vi "AlliGator Simulate Average Lifetime of Linear Combination.vi"(6 "seed":i32=-1, 8 "Error In":errorcluster, 10 "Phasor Parameters":T2, 11 "Simulation Parameters":T1) -> (0 "Error Out":errorcluster, 1 "Average Lifetimes SDV (AlliGator)":dbl[](array[numeric]), 2 "Average Lifetimes (AlliGator)":dbl[](array[numeric]), 3 "Average Lifetimes (Pure Poisson)":dbl[](array[numeric]), 4 "Message":string)   [LabVIEW 2021, in "AlliGator Shot Noise Influence on Average Lifetime.lvlib"]
doc: "Performs the simulations used in the Shot Noise Influence on Average Lifetime tool."
uses:
  AlliGator Shot Noise Influence on Average Lifetime.lvlib
  AlliGator Phasor Simulation Parameters.ctl
  AlliGator Statistics Simulation Parameters.ctl
  Histograms/Linear Histogram Options.ctl
  Histograms/Histogram Bin Option.ctl
  Histograms/Histogram Bin Position.ctl
  Phasor/Phasor Standard Deviation Options.ctl
  31c4b014-1b65-420e-a38b-b52167726bae.vi
  68577856-4cee-4ba6-b73b-a44c9001cbe5.vi
  bd7c4987-2098-4f57-a2c0-f8c7a02182c5.vi
  465ebc7b-c58a-47d8-872f-cf9e5fe3166b.vi
  bd7c4987-2098-4f57-a2c0-f8c7a02182c5.vi/e021cd17-e000-4244-b7f4-ec50548bdfcb.vi
  bd7c4987-2098-4f57-a2c0-f8c7a02182c5.vi/b1828c6e-eb0a-43e9-a724-8b596c52e435.vi
  bd7c4987-2098-4f57-a2c0-f8c7a02182c5.vi/7a6138ed-c001-4311-b538-9ba42ae7c7b1.vi
  bd7c4987-2098-4f57-a2c0-f8c7a02182c5.vi/52c6b4fa-501b-4af0-803b-8bab516ca5d3.vi
  bd7c4987-2098-4f57-a2c0-f8c7a02182c5.vi/d7237e10-35ab-4bcb-a0c6-4883c3f4c990.vi
  bd7c4987-2098-4f57-a2c0-f8c7a02182c5.vi/5fb5dd96-3b97-4592-ba56-58181c8e7105.vi
  bd7c4987-2098-4f57-a2c0-f8c7a02182c5.vi/8e13a849-a393-4484-9968-4af7b25c38d7.vi
  AlliGator Abort.vi
  <userlib>/_OpenG.lib/array/array.llb/Filter 1D Array__ogtk.vi
  <userlib>/_OpenG.lib/array/array.llb/Filter 1D Array (DBL)__ogtk.vi
  <userlib>/_OpenG.lib/array/array.llb/Delete Elements from Array__ogtk.vi
  <userlib>/_OpenG.lib/array/array.llb/Delete Elements from 1D Array (DBL)__ogtk.vi
  <vilib>/Utility/error.llb/Error Cluster From Error Code.vi
  Phasor/Phasor.lvlib
  Histograms/Histogram Window.lvlib
  Math/Math.lvlib
  GUI/GUI.lvlib
  AlliGator Globals, Variables & Constants.lvlib
  Time/Time.lvlib
  Variant/Variant.lvlib
  Utilities/Utilities.lvlib
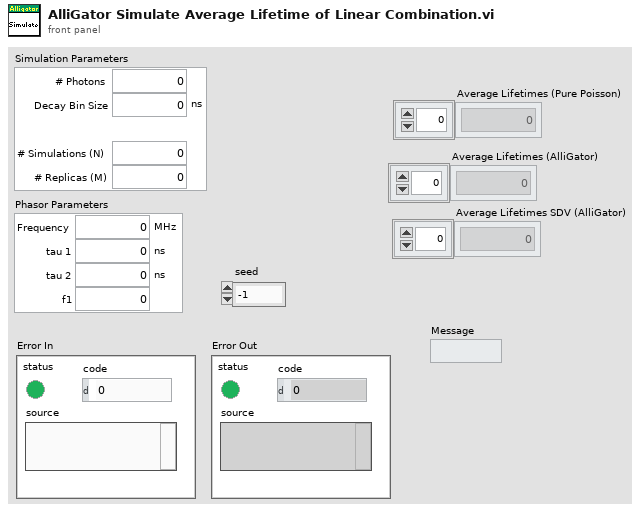
[diagram p1: front panel]
types:
  T1 = typedef "AlliGator Shot Noise Influence on Average Lifetime.lvlib/AlliGator Statistics Simulation Parameters.ctl" = cluster{"# Photons":i32, "# Replicas (M)":i32, "# Simulations (N)":i32, "Decay Bin Size":dbl[unit]}
  T2 = typedef "AlliGator Shot Noise Influence on Average Lifetime.lvlib/AlliGator Phasor Simulation Parameters.ctl" = cluster{"tau 1":dbl[unit], "tau 2":dbl[unit], "f1":dbl, "Frequency":dbl[unit]}
  T3 = typedef "Phasor.lvlib/Phasor Standard Deviation Options.ctl" = cluster{"Compute Estimated SDV":bool, "# Replicas":u32, "Use Estimated Average Phasor":bool}
  T4 = typedef "Histogram Window.lvlib/Linear Histogram Options.ctl" = cluster{"Bin Size":dbl, "Bin Number":i32, "Bin Option":T5, "Min Value":dbl, "Max Value":dbl, "Filter NaN & Infinite Values":bool, "Frequency Plot":bool, "Align Bins":bool, "Bin Location":T6, "Project Outside Values":bool, "Max Histogram Size":i32}
  T5 = typedef "Histogram Window.lvlib/Histogram Bin Option.ctl" = enum32{"Bin Number", "Bin Size"}
  T6 = typedef "Histogram Window.lvlib/Histogram Bin Position.ctl" = enum16{"Left", "Center", "Right"}
  T7 = typedef "Phasor.lvlib/Phasor (g, s).ctl" = cluster{"g":dbl, "s":dbl}
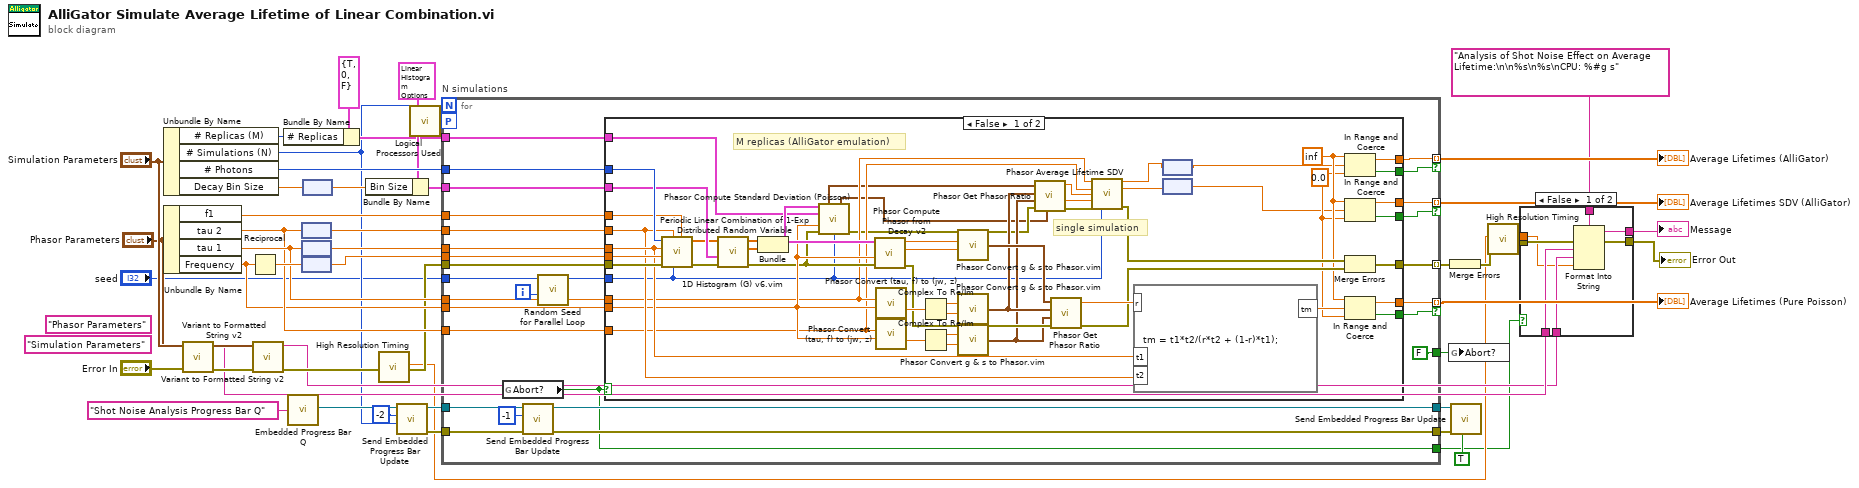
[diagram p0: block diagram]
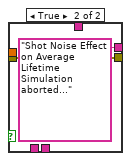
[diagram p2: hidden frame]
diagram:
  (unwired) "Phasor Parameters" ("Label")
  (unwired) "Simulation Parameters" ("Label")
  n1 = Unbundle By Name("Simulation Parameters") -> ("# Replicas (M)"=w35:i32, "# Simulations (N)"=w2:i32, "# Photons"=w48:i32, "Decay Bin Size"=w33:dbl[unit])
  n2 = Unbundle By Name("Phasor Parameters") -> ("f1"=w43:dbl, "tau 2"=w41:dbl[unit], "tau 1"=w42:dbl[unit], "Frequency"=w38:dbl[unit])
  n3 = call "Variant to Formatted String v2.vi"("error in (no error)"="Error In", "Anything"="Simulation Parameters") -> ("error out"=w15:errorcluster, "String"=w11:string)  [unwired: 8 in]
  n4 = Reciprocal(x=w38) -> (1/x=w47:dbl[unit])
  n5 = call "Variant to Formatted String v2.vi"("error in (no error)"=w15, "Anything"="Phasor Parameters") -> ("error out"=w14:errorcluster, "String"=w10:string)  [unwired: 8 in]
  n6 = Bundle By Name(cluster=T3 {"Compute Estimated SDV"=TRUE, "# Replicas"=0, "Use Estimated Average Phasor"=FALSE} ("Phasor SDV Options in"), "# Replicas"=w35) -> (w36:T3)
  n7 = call "Embedded Progress Bar Q.vi"("Progress Bar Queue Name"="Shot Noise Analysis Progress Bar Q") -> ("Progress Bar Queue"=w29:refnum<queue>)  [unwired: 6 in]
  n8 = node(w41) -> (w39:dbl)
  n9 = node(w42) -> (w40:dbl)
  n10 = node(w47) -> (w46:dbl)
  n11 = node(w33) -> (w32:dbl)
  n12 = Bundle By Name(cluster=T4 {"Bin Size"=nan, "Bin Number"=0, "Bin Option"=enum."Bin Size", "Min Value"=-inf, "Max Value"=inf, "Filter NaN & Infinite Values"=TRUE, "Frequency Plot"=FALSE, "Align Bins"=TRUE, "Bin Location"=enum."Left", "Project Outside Values"=FALSE, "Max Histogram Size"=100000} ("Histogram Options"), "Bin Size"=w32) -> (w44:T4)
  n13 = call "High Resolution Timing.vi"("Error In"=w14) -> ("elapsed (relative) seconds"=w6:dbl, "Error Out"=w8:errorcluster)  [unwired: 16 in, 1 out]
  n14 = call "Send Embedded Progress Bar Update.vi"("Max Iterations N"=w2, "Current Iteration i (i or -1: standard or || iteration; 0 or -2: first standard or || iteration)"=-2 ("Current Iteration i (-1: || iteration, -2: first || iteration)"), "Progress Bar Queue in"=w29) -> ("Error Out"=w26:errorcluster, "Progress Bar Queue out"=w28:refnum<queue>)  [unwired: 7 in]
  n15 = call "Logical Processors Used.vi"() -> ("# Logical Processor Used"=w3:i32)  [unwired: 6 in]
  n16 = for "N simulations" {
    N: w2 -> [_]
    tunnel: w48 -> [w76]
    tunnel: w46 -> [w75]
    tunnel: w8 -> [w74]
    tunnel: w44 -> [w73]
    tunnel: w43 -> [w72]
    tunnel: w42 -> [w67]
    tunnel: w41 -> [w66]
    tunnel: w38 -> [w68]
    tunnel: w40 -> [w71]
    tunnel: w39 -> [w70]
    tunnel: [w56] -> w22 mode=indexing if=w55
    tunnel: w36 -> [w69]
    tunnel: [w59] -> w23 mode=indexing if=w53
    tunnel: [w58] -> w24 mode=indexing if=w57
    tunnel: [w65] -> w34 mode=indexing
    tunnel: w26 -> [w61]
    tunnel: [w60] -> w25
    tunnel: [FALSE ("Abort?")] -> w20
    tunnel: w28 -> [w63]
    tunnel: [w62] -> w27
    workers-P: w3 -> [_]
    tunnel: [w52] -> w4
    tunnel: "seed" -> [w50]
    i -> [w51]
    n17 = global read "AlliGator Abort.vi" "Abort?"() -> (w52:bool)
    n18 = call "Send Embedded Progress Bar Update.vi"("Error In"=w61, "Current Iteration i (i or -1: standard or || iteration; 0 or -2: first standard or || iteration)"=-1 ("Current Iteration i (i or -1: standard or || iteration; 0 or -2: first standard or || iteration)"), "Progress Bar Queue in"=w63) -> ("Error Out"=w60:errorcluster, "Progress Bar Queue out"=w62:refnum<queue>)  [unwired: 7 in]
    n19 = call "Random Seed for Parallel Loop.vi"("Iteration"=w51, "Seed in (-1)"=w50) -> ("Seed out"=w49:i32)  [unwired: 9 in]
    n20 = case shown="False" w52 {
      tunnel: w76 -> [w129 _]
      tunnel: w75 -> [w128 _]
      tunnel: w74 -> [w127 w130]
      tunnel: w73 -> [w126 _]
      tunnel: w72 -> [w122 _]
      tunnel: w71 -> [w111 _]
      tunnel: w70 -> [w110 _]
      tunnel: w69 -> [w108 _]
      tunnel: w68 -> [w107 _]
      tunnel: w67 -> [w100 _]
      tunnel: w66 -> [w99 _]
      tunnel: [w94 w130] -> w65
      tunnel: [w93 _] -> w59
      tunnel: [w92 _] -> w58
      tunnel: [w91 _] -> w57
      tunnel: [w87 _] -> w56
      tunnel: [w86 _] -> w55
      tunnel: [w79 _] -> w53
      tunnel: w49 -> [w77 _]
      frame False {
        w89 = inf ("upper limit")
        w88 = 0.0 ("lower limit")
        # "M replicas (AlliGator emulation)"
        # "single simulation"
        n21 = call "Periodic Linear Combination of 1-Exp Distributed Random Variable.vi"("a 1 (in [0, 1])"=w122, "seed (-1)"=w77, "tau 2"=w110, "Error In"=w127, "T"=w128, "tau 1"=w111, "# Elements"=w129) -> ("Error Out"=w125:errorcluster, "t Array"=w78:dbl[])  [unwired: 3 in]
        n22 = call "1D Histogram (G) v6.vim"("Error In"=w125, "Histogram Options"=w126, "Array"=w78) -> ("Error Out"=w105:errorcluster, "Histogram"=w123:dbl[], "Axis"=w124:dbl[])  [unwired: 2 in, 4 out]
        n23 = Bundle("Axis"=w124, "Histogram"=w123) -> (w109:cluster{"Axis":dbl[], "Histogram":dbl[]})  [unwired: 1 in]
        n24 = call "Phasor Compute Standard Deviation (Poisson).vi"("Time-Gated Decay"=w109, "Phasor SDV Options in"=w108, "Phasor Frequency"=w107, "Error In"=w105, "seed"=w77) -> ("(Mean) Phasor (g, s)"=w81:T7, "Phasor SDV (g, s)"=w80:T7, "Error Out"=w97:errorcluster)  [unwired: 4 in, 4 out]
        n25 = call "Phasor Compute Phasor from Decay v2.vi"("Error In"=w105, "Phasor Frequency"=w107, "Time-Gated Decay"=w109) -> ("Error Out"=w106:errorcluster, "s"=w113:dbl, "g"=w114:dbl)  [unwired: 5 in, 1 out]
        n26 = call "Phasor Convert (tau, f) to (jw, z).vi"("Harmonic Frequency"=w107, "Lifetime"=w100) -> ("Phasor"=w121:cdb)  [unwired: 8 in, 1 out]
        n27 = call "Phasor Convert (tau, f) to (jw, z).vi"("Harmonic Frequency"=w107, "Lifetime"=w99) -> ("Phasor"=w116:cdb)  [unwired: 8 in, 1 out]
        n28 = Complex To Re/Im(x + iy=w121) -> (x=w120:dbl, y=w119:dbl)
        n29 = Complex To Re/Im(x + iy=w116) -> (x=w117:dbl, y=w118:dbl)
        n30 = call "Phasor Convert g & s to Phasor.vim"("s"=w113, "g"=w114) -> ("Phasor Array"=w112:T7)  [unwired: 8 in]
        n31 = call "Phasor Convert g & s to Phasor.vim"("s"=w119, "g"=w120) -> ("Phasor Array"=w104:T7)  [unwired: 8 in]
        n32 = call "Phasor Convert g & s to Phasor.vim"("s"=w118, "g"=w117) -> ("Phasor Array"=w103:T7)  [unwired: 8 in]
        n33 = call "Phasor Get Phasor Ratio.vi"("Phasor SDV"=w80, "Error In"=w97, "Reference Phasor 2"=w103, "Reference Phasor 1"=w104, "Phasor"=w81) -> ("Error Out"=w98:errorcluster, "Phasor Ratio SDV"=w102:dbl, "Phasor Ratio (f1)"=w101:dbl)  [unwired: 4 in]
        n34 = call "Phasor Get Phasor Ratio.vi"("Error In"=w106, "Reference Phasor 2"=w103, "Reference Phasor 1"=w104, "Phasor"=w112) -> ("Error Out"=w95:errorcluster, "Phasor Ratio (f1)"=w115:dbl)  [unwired: 5 in, 1 out]
        n35 = call "Phasor Average Lifetime SDV.vi"("tau 1"=w100, "tau 2"=w99, "r"=w101, "SDV r"=w102, "Error In"=w98, "seed"=w77) -> ("<tau>_a"=w85:dbl[unit], "SDV <tau>_a"=w83:dbl[unit], "Error Out"=w96:errorcluster)  [unwired: 4 in, 3 out]
        n36 = formula code="tm = t1*t2/(r*t2 + (1-r)*t1);"("r"=w115, "t1"=w111, "t2"=w110) -> ("tm"=w90:dbl)
        n37 = node(w85) -> (w84:dbl)
        n38 = node(w83) -> (w82:dbl)
        n39 = In Range and Coerce(upper limit=w89, x=w84, lower limit=w88) -> (coerced(x)=w93:dbl, In Range?=w79:bool)
        n40 = In Range and Coerce(upper limit=w89, x=w82, lower limit=w88) -> (coerced(x)=w92:dbl, In Range?=w91:bool)
        n41 = Merge Errors(w96, w95) -> (w94:errorcluster)
        n42 = In Range and Coerce(upper limit=w89, x=w90, lower limit=w88) -> (coerced(x)=w87:dbl, In Range?=w86:bool)
      }
      frame True {
      }
    }
  }
  "Average Lifetimes (Pure Poisson)" <- w22
  "Average Lifetimes (AlliGator)" <- w23
  "Average Lifetimes SDV (AlliGator)" <- w24
  n43 = global write "AlliGator Abort.vi" "Abort?"(w20) -> ()
  n44 = Merge Errors(w34) -> (w19:errorcluster)
  n45 = call "Send Embedded Progress Bar Update.vi"("Stop Progress Bar (F)"=TRUE, "Error In"=w25, "Progress Bar Queue in"=w27) -> ()  [unwired: 7 in, 2 out]
  n46 = call "High Resolution Timing.vi"("relative seconds (NaN)"=w6, "Error In"=w19) -> ("elapsed (relative) seconds"=w5:dbl, "Error Out"=w7:errorcluster)  [unwired: 15 in, 1 out]
  n47 = case shown="False" w4 {
    tunnel: [w137 w138] -> w18
    tunnel: [w136 "Shot Noise Effect on Average Lifetime Simulation aborted..."] -> w17
    tunnel: w11 -> [w135 _]
    tunnel: w10 -> [w134 _]
    tunnel: "Analysis of Shot Noise Effect on Average Lifetime:\n\n%s\n%s\nCPU: %#g s" ("format string") -> [w133 _]
    tunnel: w7 -> [w132 w138]
    tunnel: w5 -> [w131 _]
    frame False {
      n48 = Format Into String(format string=w133, error in=w132, w135, w134, w131) -> (resulting string=w136:string, error out=w137:errorcluster)  [unwired: 1 in]
    }
    frame True {
    }
  }
  "Error Out" <- w18
  "Message" <- w17
